vi "ble_cmd_attclient_read_by_group_type.vi"(4 "Service Type (0x2800)":T1=10240 format="%04x" items=["Primary"=10240, "Secundary"=10241], 5 "Last Handle Number (0xFFFF)":u16=65535 format="%04x", 6 "Connection Status":T2={"MAC Address"="", "cnx handle"=0, "cnx flags"=0, "Address Type"=125, "Connection Interval (ms)"=125, "Timeout(ms)"=125, "Latency"=0, "bonding handle"=0} {"Address Type" items=["Public", "Random"]}, 7 "First Handle Number(0x0001)":u16=1 format="%04x", 8 "error in (no error)":errorcluster, 11 "COM Bluegiga in":refnum<visa-resource-name>) -> (0 "error out":errorcluster, 3 "COM Bluegiga out":refnum<visa-resource-name>)   [LabVIEW 2017]
uses:
  type_def/connection_status_bundle.ctl
  type_def/address_type.ctl
  type_def/service_type.ctl
  type_def/message_class.ctl
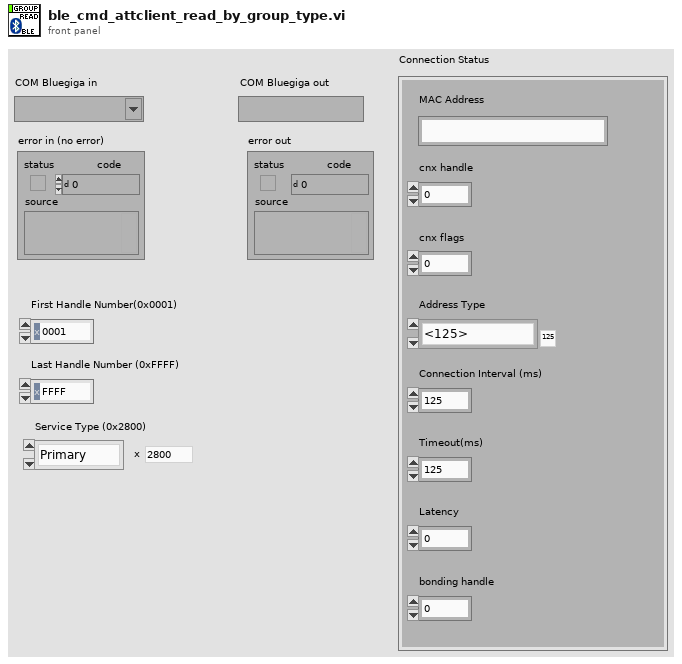
[diagram p1: front panel]
types:
  T1 = typedef "service_type.ctl" = u16
  T2 = typedef "connection_status_bundle.ctl" = cluster{"MAC Address":string, "cnx handle":u8, "cnx flags":u8, "Address Type":T3, "Connection Interval (ms)":u16, "Timeout(ms)":u16, "Latency":u16, "bonding handle":u8}
  T3 = typedef "address_type.ctl" = u8
  T4 = typedef "message_class.ctl" = u8
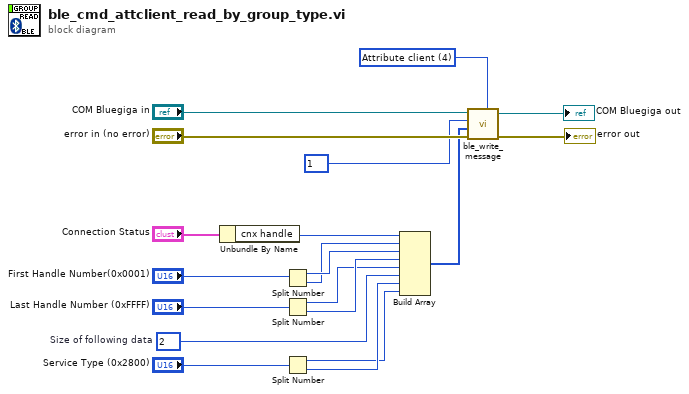
[diagram p0: block diagram]
diagram:
  w7 = u8 2  # Size of following data
  w6 = T4 4 items=["System", "Persistent Store", "Attribute database", "Connection", "Attribute client", "Security Manager", "Generic Access Profile", "Hardware"] ("Command Class (System)")
  n1 = Unbundle By Name("Connection Status") -> ("cnx handle"=w15:u8)
  n2 = Split Number(x="First Handle Number(0x0001)") -> (hi(x)=w12:u8, lo(x)=w11:u8)
  n3 = Split Number(x="Last Handle Number (0xFFFF)") -> (hi(x)=w9:u8, lo(x)=w10:u8)
  n4 = Split Number(x="Service Type (0x2800)") -> (hi(x)=w3:u8, lo(x)=w4:u8)
  n5 = Build Array(w15, w11, w12, w10, w9, w7, w4, w3) -> (w14:u8[])
  n6 = call "ble_write_message.vi"("Command Class (System)"=w6, "error in (no error)"="error in (no error)", "Payload(Empty)"=w14, "Message ID (0x00)"=u8 1, "COM Bluegiga in"="COM Bluegiga in") -> ("error out"=→"error out":errorcluster, "COM Bluegiga out"=→"COM Bluegiga out":refnum<visa-resource-name>)  [unwired: 4 in, 1 out]
